vi "ICNC Machine Home.vi"(5 "MaxStrokeB":u32, 6 "MaxStrokeA":u32, 7 "MaxStrokeZ":u32, 8 "error in (no error)":errorcluster caption="entrée d'erreur (pas d'erreur)", 9 "MaxStrokeY":u32, 10 "MaxStrokeX":u32, 11 "Axis":u32) -> (0 "error out":errorcluster caption="sortie d'erreur", 3 "function return":u32)   [LabVIEW 2012, in "ICNC2.lvlib"]
doc: "DWORD ICNC_MachineHome( DWORD Axis,\n DWORD MaxStrokeX=0xFFFFFFFF,\n DWORD MaxStrokeY=0xFFFFFFFF,\n DWORD MaxStrokeZ=0xFFFFFFFF,\n DWORD MaxStrokeA=0xFFFFFFFF,\n DWORD MaxStrokeB=0xFFFFFFFF);"
uses:
  <userlib>/ICNC/ICNC2.lvlib
  <userlib>/ICNC/ICNC2.dll
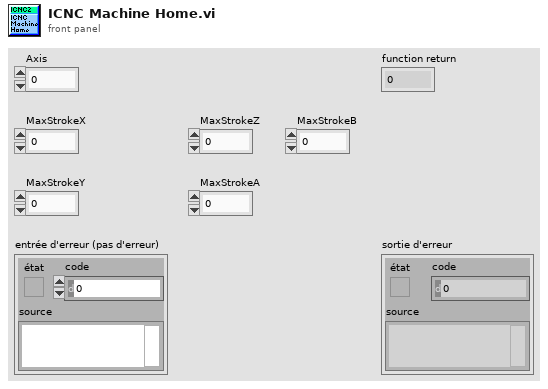
[diagram p1: front panel]
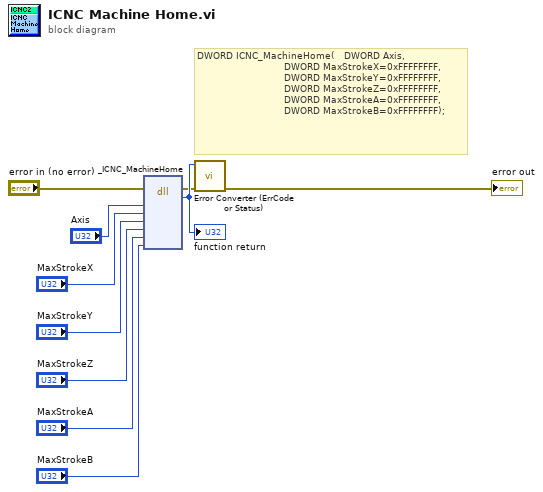
[diagram p0: block diagram]
diagram:
  # "DWORD ICNC_MachineHome(   DWORD Axis,\n                             DWORD MaxStrokeX=0xFFFFFFFF,\n                             DWORD MaxStrokeY=0xFFFFFFFF,\n                             DWORD MaxStrokeZ=0xFFFFFFFF,\n                             DWORD MaxStrokeA=0xFFFFFFFF,\n                             DWORD MaxStrokeB=0xFFFFFFFF);"
  n1 = dll-call lib="C:/Program Files (x86)/National Instruments/LabVIEW 2012/user.lib/ICNC/ICNC2.*" fn="_ICNC_MachineHome"(error in="error in (no error)", "Axis"="Axis", "MaxStrokeX"="MaxStrokeX", "MaxStrokeY"="MaxStrokeY", "MaxStrokeZ"="MaxStrokeZ", "MaxStrokeA"="MaxStrokeA", "MaxStrokeB"="MaxStrokeB") -> (error out=w2:errorcluster, w10:u32)  [unwired: 8 in, 1 out]
  "function return" <- w10
  n2 = call <userlib>:"Error Converter (ErrCode or Status).vi"("error in (no error)"=w2, "error code"=w10) -> ("error out"=→"error out":errorcluster)  [unwired: 9 in]
